vi "Build Report.vi"(5 "3rd Party Member Data":string[][](array[string]), 7 "User.lib Member Data":string[][](array[string]), 8 "error in (no error)":errorcluster, 9 "Unreferenced Files":path[](array[path]), 10 "Project Summary":T1={"Project Name"="Test Name", "Project Path"=path "C:/Projects/Project Scanner", "# VIs in Project"=6, "# VIs Unreviewed"=5, "Date of Last Review"=timestamp(3413822768.062893 s since 1904-01-01), "# of VIs without Caller"=4, "Project Description"="Test Description", "# VIs Modified"=3}, 11 "Project Member Data":string[][](array[string])) -> (0 "error out":errorcluster)   [LabVIEW 2014]
doc: "<b>Controls:</b> \n<b>Inputs:</b>\n<b>error in (no error):</b>\n<B>error in</B> can accept error information wired from VIs previously called. Use this information to decide if any functionality should be bypassed in the event of errors from other VIs.\n\nRight-click the <B>error in</B> control on the front panel and select <B>Explain Error</B> or <B>Explain Warning</B> from the shortcut menu for more information about the error. \n\n<b>Project Summary:</b>\n\n\n<b>Project Member Data:</b>\n\n\n<b>User.lib Member Data:</b>\n\n\n<b>3rd Party Member Data:</b>\n\n\n<b>Unreferenced Files:</b>\n\n\n<b>Outputs:</b>\n<b>error out:</b>\n<B>error out</B> passes error or warning information out of a VI to be used by other VIs.\n\nRight-click the <B>error out</B> indicator on the front panel and select <B>Explain Error</B> or <B>Explain Warning</B> from the shortcut menu for more information about the error."
uses:
  Type Defs/TYPE_Project Summary.ctl
  <vilib>/Utility/NIReport.llb/NI_report.lvclass
  <vilib>/Utility/NIReport.llb/Excel/NI_Excel.lvclass
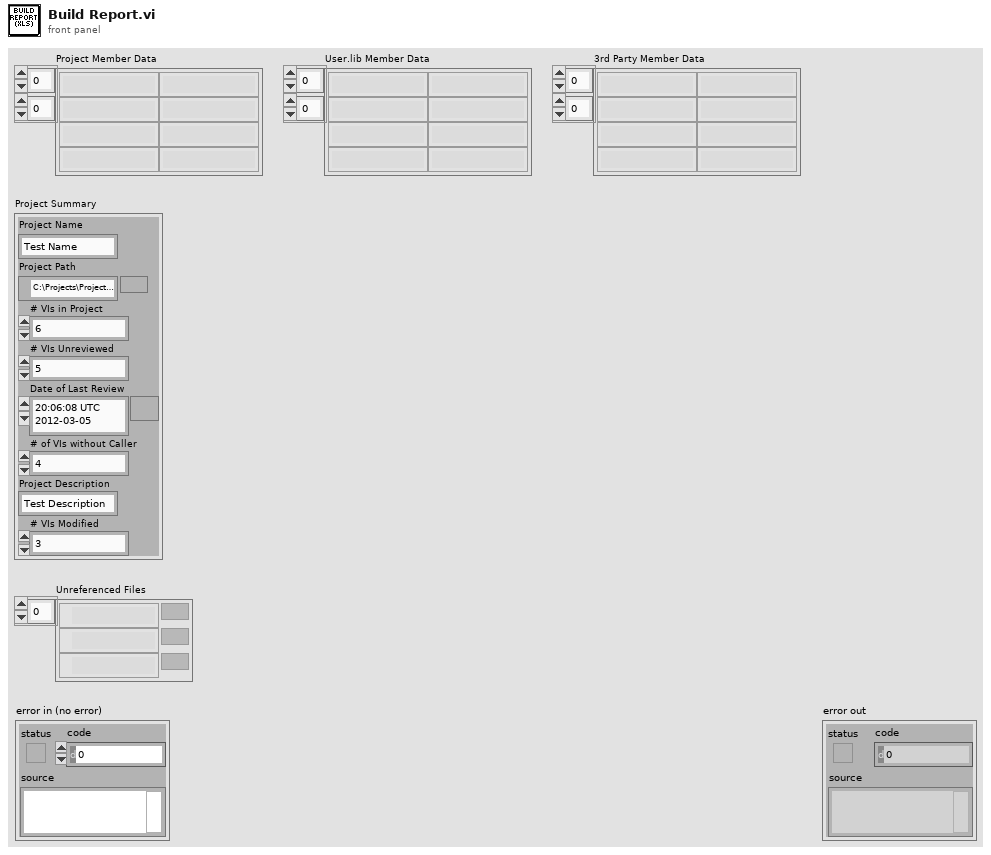
[diagram p1: front panel]
types:
  T1 = typedef "TYPE_Project Summary.ctl" = cluster{"Project Name":string, "Project Path":path, "# VIs in Project":i32, "# VIs Unreviewed":i32, "Date of Last Review":timestamp, "# of VIs without Caller":i32, "Project Description":string, "# VIs Modified":i32}
  T2 = enum16{"Standard Report", "HTML", "Word", "Excel"}
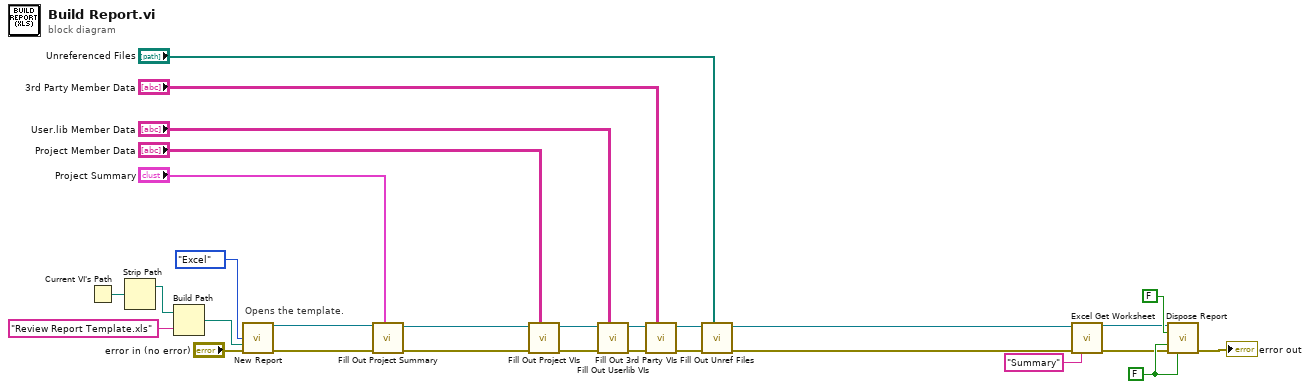
[diagram p0: block diagram]
diagram:
  w20 = FALSE ("save changes? (F)")
  # "Opens the template."
  n1 = Current VI's Path() -> (path=w26:path)
  n2 = Strip Path(path=w26) -> (stripped path=w28:path)  [unwired: 1 out]
  n3 = Build Path(base path=w28, name or relative path="Review Report Template.xls") -> (appended path=w25:path)
  n4 = call <vilib>:"New Report.vi"("report type"=T2."Excel", "template (empty)"=w25, "error in (no error)"="error in (no error)") -> ("report out"=w23:refnum<class "NI_report.lvclass">, "error out"=w22:errorcluster)  [unwired: 11 in]
  n5 = call "Fill Out Project Summary.vi"("Project Summary"="Project Summary", "error in (no error)"=w22, "NI_report in"=w23) -> ("error out"=w16:errorcluster, "NI_report out"=w17:refnum<class "NI_report.lvclass">)  [unwired: 7 in]
  n6 = call "Fill Out Project VIs .vi"("Project Member Data"="Project Member Data", "error in (no error)"=w16, "NI_report in"=w17) -> ("error out"=w11:errorcluster, "NI_report out"=w12:refnum<class "NI_report.lvclass">)  [unwired: 7 in]
  n7 = call "Fill Out Userlib VIs .vi"("user.lib Member Data"="User.lib Member Data", "error in (no error)"=w11, "NI_report in"=w12) -> ("error out"=w9:errorcluster, "NI_report out"=w10:refnum<class "NI_report.lvclass">)  [unwired: 7 in]
  n8 = call "Fill Out 3rd Party VIs .vi"("3rd Party Member Data"="3rd Party Member Data", "error in (no error)"=w9, "NI_report in"=w10) -> ("error out"=w1:errorcluster, "NI_report out"=w5:refnum<class "NI_report.lvclass">)  [unwired: 7 in]
  n9 = call "Fill Out Unref Files.vi"("Unreferenced Files"="Unreferenced Files", "error in (no error)"=w1, "NI_report in"=w5) -> ("error out"=w2:errorcluster, "NI_report out"=w3:refnum<class "NI_report.lvclass">)  [unwired: 7 in]
  n10 = call <vilib>:"Excel Get Worksheet.vi"("report in"=w3, "error in (no error)"=w2, "name (\"\")"="Summary" ("name (\"\")")) -> ("report out"=w15:refnum<class "NI_report.lvclass">, "error out"=w14:errorcluster)  [unwired: 11 in]
  n11 = call-dynamic "Dispose Report.vi"("report in"=w15, "wait until printing completed? (T)"=FALSE, "save changes? (F)"=w20, "error in (no error)"=w14, "close report? (T)"=w20) -> ("error out"=→"error out":errorcluster)  [unwired: 10 in]
